vi "remove-edge-from-pred-and-succ-maps.vi"(8 "sink-id":refnum<class "ID.lvclass">, 9 "source-id":refnum<class "ID.lvclass">, 10 "node-successors-by-id":T1(c390), 11 "node-predecessors-by-id":T1(c390)) -> (2 "node-successors-by-id out":T1(c390), 3 "node-predecessors-by-id out":T1(c390))   [LabVIEW 2020, in "graph.lvlib" / "DiGraph.lvclass"]
uses:
  DiGraph.lvclass
  ID/ID.lvclass
  62745b6b-b1f0-4e9a-9807-6e89714fdb4f.vi
  b8df6df7-5257-4220-8012-abd1467aebb7.vi
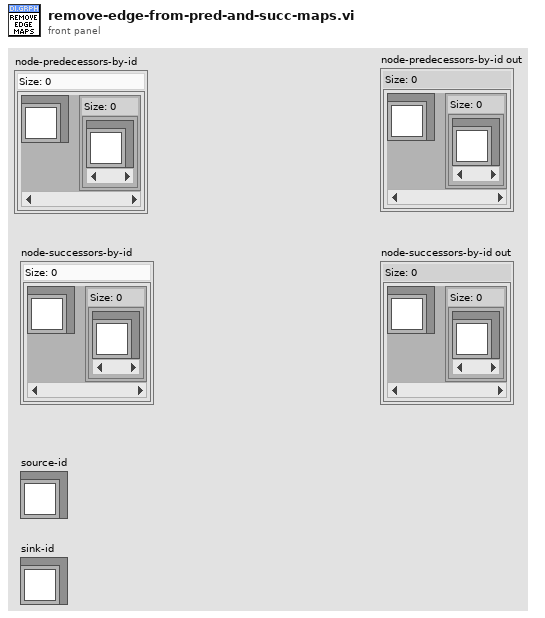
[diagram p1: front panel]
types:
  T1 = map{refnum<class "ID.lvclass">, set{refnum<class "ID.lvclass">}}
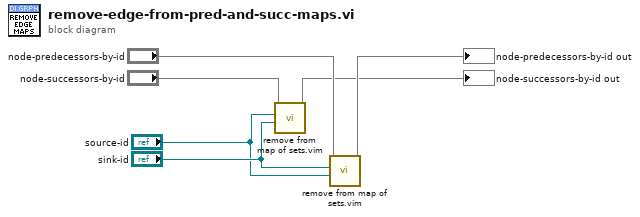
[diagram p0: block diagram]
diagram:
  n1 = call "remove from map of sets.vim"("value"="sink-id", "key"="source-id", "map of sets in"="node-successors-by-id") -> ("map of sets out"=→"node-successors-by-id out":T1)  [unwired: 6 in, 2 out]
  n2 = call "remove from map of sets.vim"("value"="source-id", "key"="sink-id", "map of sets in"="node-predecessors-by-id") -> ("map of sets out"=→"node-predecessors-by-id out":T1)  [unwired: 6 in, 2 out]
